vi "ShooterOutput.vi"() -> ()   [LabVIEW 2019]
uses:
  <vilib>/Rock Robotics/WPI/ThirdParty/REV Robotics/SPARK MAX/Typedef/Spark MAX Control Type.ctl
  <vilib>/Rock Robotics/WPI/Solenoid/WPI_SolenoidValue.ctl
  967c0bfc-6427-4b0b-9d33-318ccee3f8f4.vi
  ee6d7eed-3121-4b7e-b0b1-4827d4be6c14.vi
  refnums.vi
  GRNF_GenericMotor.vi
  GRNF_GenericSolenoid.vi
  sensors.vi
  outputs.vi
  dsdata.vi
  <vilib>/Rock Robotics/WPI/Solenoid/WPI_SolenoidSetEnum.vi
panel:
  in  "Plot Kicker":bool
  out "Kicker":T1(graph)
  in  "Kicker PID":T2={"P Gain"=0.0001, "I Gain"=1e-07, "D Gain"=0.01, "F Gain"=0.0002, "I Zone"=200.0, "Min Output"=0.0, "Max Output"=1.0} {"Max Output" min=-1.0 max=1.0 step=0.01; "Min Output" min=-1.0 max=1.0 step=0.01; "I Zone" step=0.01; "F Gain" step=0.01; "D Gain" step=0.01; "I Gain" step=0.01; "P Gain" min=0.0 step=0.01}
  out "Shooter 1":T1(graph)
  in  "Plot Shooter":bool
  out "Shooter 0":T1(graph)
  in  "Shooter PID":T2={"P Gain"=0.0027, "I Gain"=0.0, "D Gain"=0.007, "F Gain"=0.00017, "I Zone"=200.0, "Min Output"=0.0, "Max Output"=1.0} {"Max Output" min=-1.0 max=1.0 step=0.01; "Min Output" min=-1.0 max=1.0 step=0.01; "I Zone" step=0.01; "F Gain" step=0.01; "D Gain" step=0.01; "I Gain" step=0.01; "P Gain" min=0.0 step=0.01}
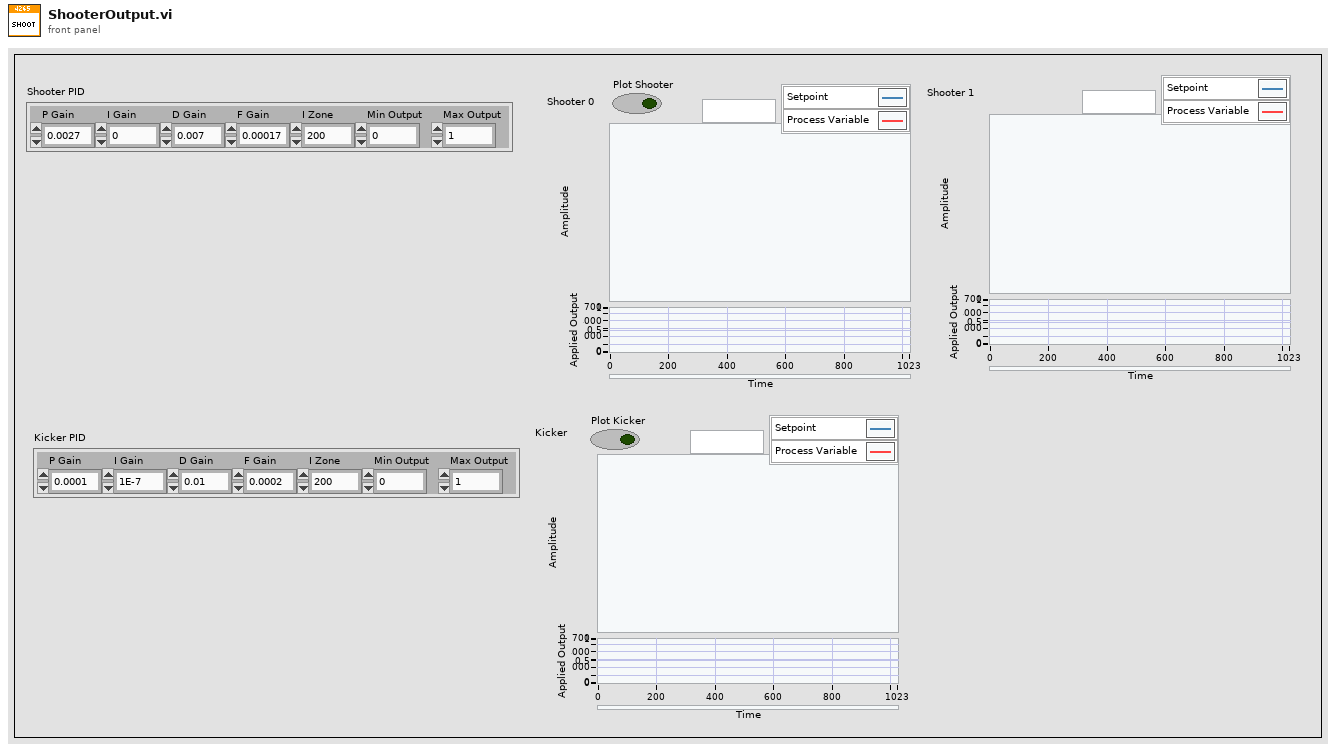
[diagram p1: front panel]
types:
  T1 = cluster{"Sensor Velocity":dbl, "Setpoint":dbl, "Applied Output":dbl}
  T2 = cluster{"P Gain":dbl, "I Gain":dbl, "D Gain":dbl, "F Gain":dbl, "I Zone":dbl, "Min Output":dbl, "Max Output":dbl}
  T3 = typedef "Spark MAX Control Type.ctl" = enum16{"Percent VBus", "Voltage", "Velocity", "Position", "Smart Motion", "Current", "Smart Velocity"}
  T4 = typedef "WPI_MotorControlDeviceRef.ctl" = cluster{"DeviceStatus":errorcluster, "Type":T5, "PWM":cluster{"PWM Channel":T6, "DeadBand":T7}, "CAN":cluster{"Device Number":u8, "SetOutput VI Ref":variant, "GetOutput VI Ref":variant, "Enable VI Ref":variant, "Disable VI Ref":variant, "Data":variant}, "Invert":bool, "DIO PWM":cluster{"PWM \"Enable\" Channel":T6, "DIOChannel":T8, "PWM Rate":dbl}}
  T5 = typedef "WPI_MotorControlType.ctl" = enum16{"PWM", "CAN", "DIO PWM"}
  T6 = typedef "FPGA_DIOPWMChannel.ctl" = enum8{"PWM 0", "PWM 1", "PWM 2", "PWM 3", "PWM 4", "PWM 5", "PWM 6", "PWM 7", "PWM 8", "PWM 9", "PWM MXP 0", "PWM MXP 1", "PWM MXP 2", "PWM MXP 3", "PWM MXP 4", "PWM MXP 5", "PWM MXP 6", "PWM MXP 7", "PWM MXP 8", "PWM MXP 9", "Invalid"}
  T7 = typedef "WPI_PWMDeadband.ctl" = cluster{"Name":string, "maxPositivePwm":i32, "minPositivePwm":i32, "centerPwm":i32, "maxNegativePwm":i32, "minNegativePwm":i32, "angularRange":u16}
  T8 = typedef "FPGA_DIOChannel.ctl" = enum8{"DIO 0", "DIO 1", "DIO 2", "DIO 3", "DIO 4", "DIO 5", "DIO 6", "DIO 7", "DIO 8", "DIO 9", "DIO MXP 0", "DIO MXP 1", "DIO MXP 2", "DIO MXP 3", "DIO MXP 4", "DIO MXP 5", "DIO MXP 6", "DIO MXP 7", "DIO MXP 8", "DIO MXP 9", "DIO MXP 10", "DIO MXP 11", "DIO MXP 12", "DIO MXP 13", "DIO MXP 14", "DIO MXP 15", "SPI Port CS1", "SPI Port CS2", "SPI Port CS3", "SPI Port MISO", "SPI Port MOSI", "Invalid"}
  T9 = typedef "WPI_SolenoidDevRef.ctl" = cluster{"DevStatus":errorcluster, "Pneumatics Control Module":u8, "Forward Solenoid Channel":T10, "Reverse Solenoid Channel":T10}
  T10 = typedef "WPI_SolenoidChannel.ctl" = enum8{"Solenoid 0", "Solenoid 1", "Solenoid 2", "Solenoid 3", "Solenoid 4", "Solenoid 5", "Solenoid 6", "Solenoid 7", "Invalid"}
  T11 = typedef "WPI_DriverStationRobotMode2.ctl" = enum16{"Autonomous Disabled", "Autonomous Enabled", "Teleop Disabled", "Teleop Enabled", "Disconnected", "Finish", "Test Disabled", "Test Enabled", "Emergency Stopped"}
  T12 = cluster{"P Gain":bool, "I Gain":bool, "D Gain":bool, "F Gain":bool, "I Zone":bool, "Min Output":bool, "Max Output":bool}
  T13 = typedef "WPI_SolenoidValue.ctl" = enum16{"Off", "On", "Forward", "Reverse"}
  T14 = cluster{"Goal_Kicker_Speed (rpm)":dbl, "Kicker_Velocity (rpm)":dbl, "Applied Output":dbl}
  T15 = cluster{"Goal_Shooter_Speed (rpm)":dbl, "Shooter_0_Velocity (rpm)":dbl, "Applied Output":dbl}
  T16 = cluster{"Goal_Shooter_Speed (rpm)":dbl, "Shooter_1_Velocity (rpm)":dbl, "Applied Output":dbl}
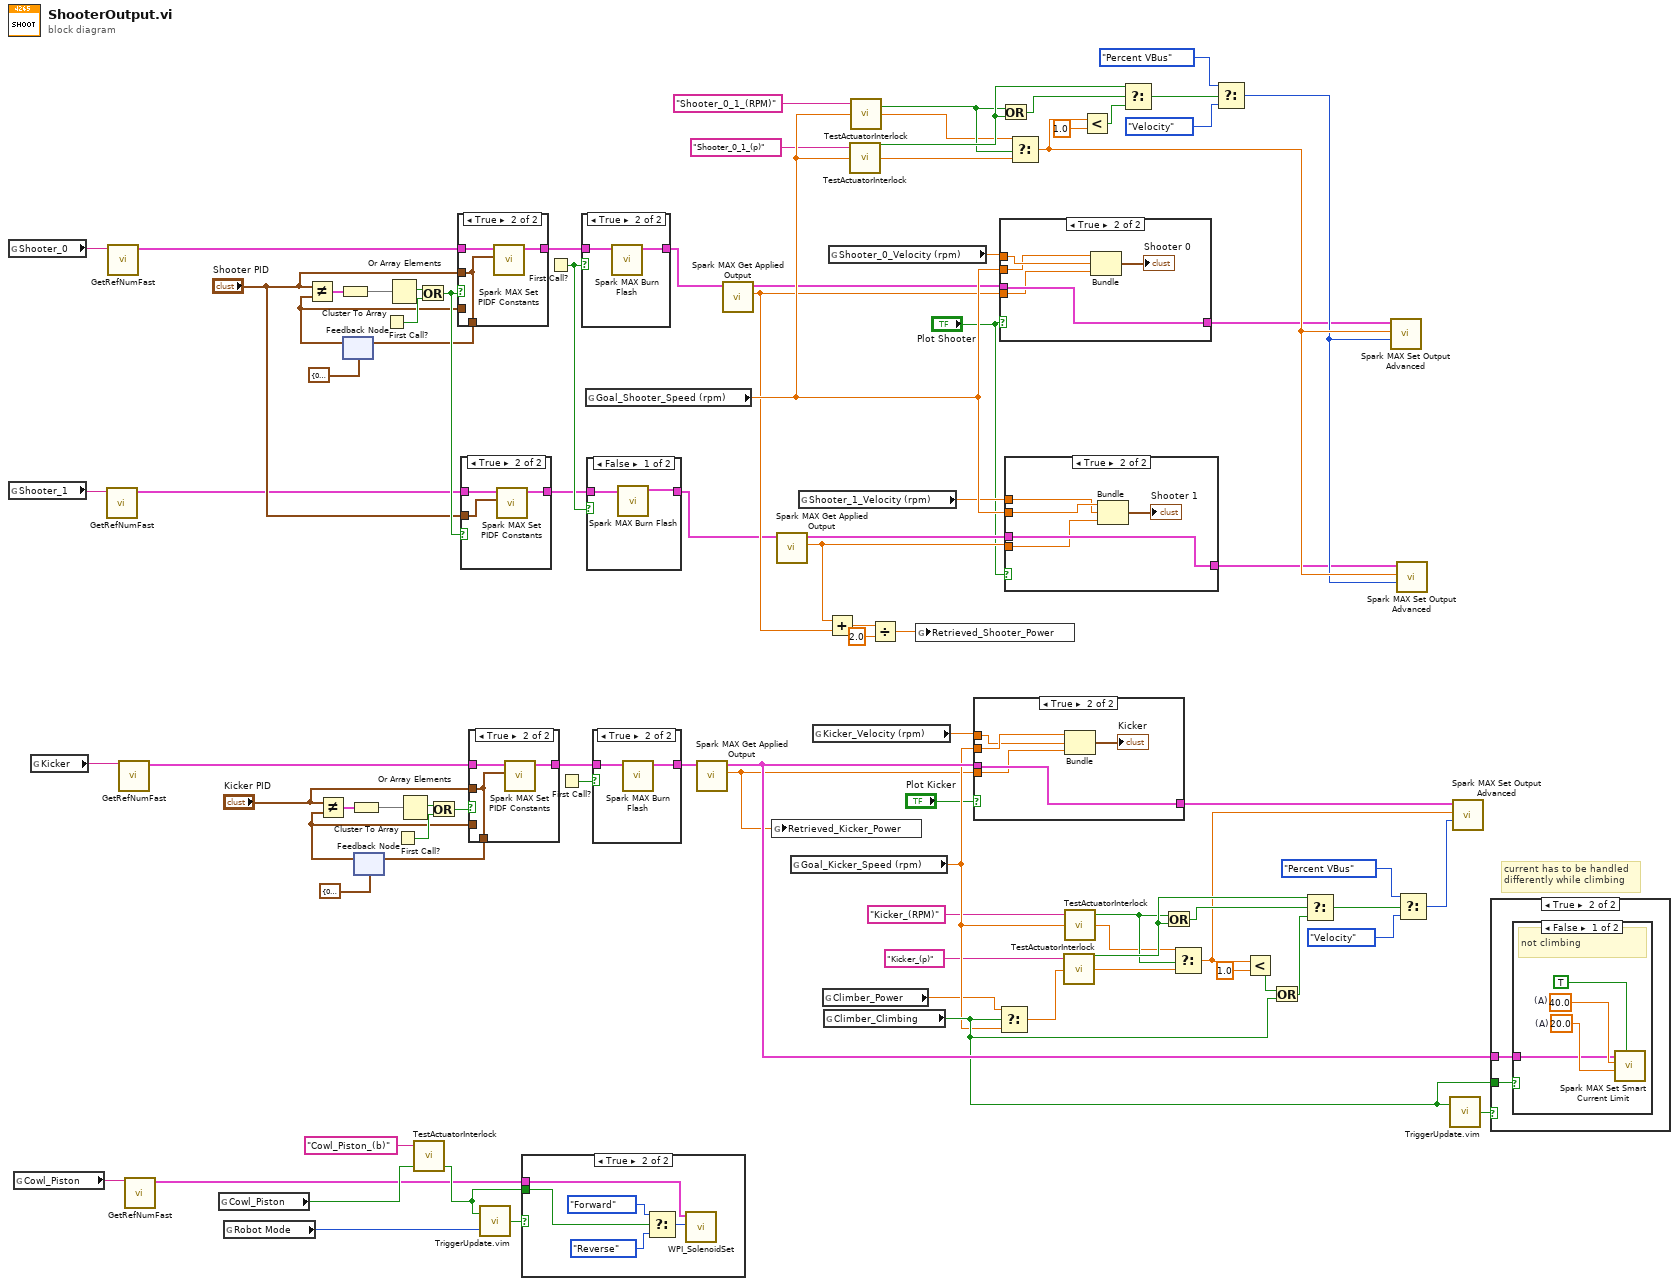
[diagram p0: block diagram]
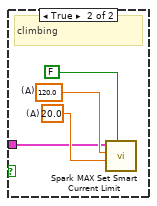
[diagram p3: hidden frame]
diagram:
  # "current has to be handled\ndifferently while climbing"
  n1 = global read "refnums.vi" "Shooter_0"() -> (w4:string)
  n2 = global read "refnums.vi" "Shooter_1"() -> (w3:string)
  n3 = global read "refnums.vi" "Cowl_Piston"() -> (w1:string)
  n4 = global read "refnums.vi" "Kicker"() -> (w2:string)
  n5 = call-poly "GetRefNumFast.vi"("RefNum Name"=w3) -> ("Device Reference"=w7:T4)  [unwired: 5 in, 1 out]
  n6 = call-poly "GetRefNumFast.vi"("RefNum Name"=w4) -> ("Device Reference"=w8:T4)  [unwired: 5 in, 1 out]
  n7 = call-poly "GetRefNumFast.vi"("RefNum Name"=w2) -> ("Device Reference"=w6:T4)  [unwired: 5 in, 1 out]
  n8 = call-poly "GetRefNumFast.vi"("RefNum Name"=w1) -> ("Device Reference"=w5:T9)  [unwired: 5 in, 1 out]
  n9 = global read "outputs.vi" "Cowl_Piston"() -> (w58:bool)
  n10 = global read "dsdata.vi" "Robot Mode"() -> (w35:T11)
  n11 = feedback #1(T2 {"P Gain"=0.0, "I Gain"=0.0, "D Gain"=0.0, "F Gain"=0.0, "I Zone"=0.0, "Min Output"=0.0, "Max Output"=0.0} ("PID Constants")) -> (w9:T2)
  n12 = Not Equal?(x="Shooter PID", y=w9) -> (x != y?=w13:T12)
  n13 = Cluster To Array(cluster=w13) -> (array=w12:bool[])
  n14 = feedback #2(T2 {"P Gain"=0.0, "I Gain"=0.0, "D Gain"=0.0, "F Gain"=0.0, "I Zone"=0.0, "Min Output"=0.0, "Max Output"=0.0} ("PID Constants")) -> (w37:T2)
  n15 = Not Equal?(x="Kicker PID", y=w37) -> (x != y?=w41:T12)
  n16 = Cluster To Array(cluster=w41) -> (array=w40:bool[])
  n17 = First Call?() -> (First Call?: T/F=w16:bool)
  n18 = Or Array Elements(Boolean array=w12) -> (logical OR=w15:bool)
  n19 = First Call?() -> (First Call?: T/F=w44:bool)
  n20 = Or Array Elements(Boolean array=w40) -> (logical OR=w43:bool)
  n21 = call "TestActuatorInterlock.vi"("Input_Value_Boolean"=w58, "Actuator_Name"="Cowl_Piston_(b)") -> ("Output_Value_Boolean"=w59:bool)  [unwired: 1 in, 2 out]
  n22 = Or(x=w15, y=w16) -> (x .or. y?=w19:bool)
  n23 = Or(x=w43, y=w44) -> (x .or. y?=w46:bool)
  n24 = case shown="True" w19 {
    tunnel: w8 -> [w92 w96]
    tunnel: "Shooter PID" -> [_ w94]
    tunnel: [w93 w94] -> w10
    tunnel: w9 -> [w93 _]
    tunnel: [w92 w95] -> w14
    frame False {
    }
    frame True {
      n25 = call <vilib>:"Spark MAX Set PIDF Constants.vi"("PID Constants"=w94, "MotorControlDeviceRef"=w96) -> ("MotorControlDeviceRef"=w95:T4)  [unwired: 8 in, 1 out]
    }
  }
  n26 = feedback-in #1(w10) -> ()
  n27 = case shown="True" w19 {
    tunnel: w7 -> [w97 w100]
    tunnel: "Shooter PID" -> [_ w98]
    tunnel: [w97 w99] -> w17
    frame False {
    }
    frame True {
      n28 = call <vilib>:"Spark MAX Set PIDF Constants.vi"("PID Constants"=w98, "MotorControlDeviceRef"=w100) -> ("MotorControlDeviceRef"=w99:T4)  [unwired: 8 in, 1 out]
    }
  }
  n29 = case shown="True" w46 {
    tunnel: w6 -> [w101 w105]
    tunnel: "Kicker PID" -> [_ w103]
    tunnel: [w102 w103] -> w38
    tunnel: w37 -> [w102 _]
    tunnel: [w101 w104] -> w42
    frame False {
    }
    frame True {
      n30 = call <vilib>:"Spark MAX Set PIDF Constants.vi"("PID Constants"=w103, "MotorControlDeviceRef"=w105) -> ("MotorControlDeviceRef"=w104:T4)  [unwired: 8 in, 1 out]
    }
  }
  n31 = feedback-in #2(w38) -> ()
  n32 = call "TriggerUpdate.vim"("Robot Mode"=w35, "Trigger"=w59) -> ("Update"=w36:bool)
  n33 = case shown="True" w36 {
    tunnel: w59 -> [_ w106]
    tunnel: w5 -> [_ w107]
    frame False {
    }
    frame True {
      n34 = Select(t=WPI_SolenoidValue."Forward" ("Value"), s=w106, f=WPI_SolenoidValue."Reverse" ("Value")) -> (s? t:f=w110:T13)
      n35 = call-poly <vilib>:"WPI_SolenoidSet.vi"("Value"=w110, "SolenoidDevRef"=w107) -> ()  [unwired: 8 in, 2 out]
    }
  }
  n36 = First Call?() -> (First Call?: T/F=w20:bool)
  n37 = First Call?() -> (First Call?: T/F=w47:bool)
  n38 = case shown="True" w20 {
    tunnel: w14 -> [w111 w113]
    tunnel: [w111 w112] -> w26
    frame False {
    }
    frame True {
      n39 = call <vilib>:"Spark MAX Burn Flash.vi"("MotorControlDeviceRef"=w113) -> ("MotorControlDeviceRef"=w112:T4)  [unwired: 9 in, 1 out]
    }
  }
  n40 = global read "outputs.vi" "Goal_Shooter_Speed (rpm)"() -> (w81:dbl)
  n41 = case shown="False" w20 {
    tunnel: [w114 w116] -> w28
    tunnel: w17 -> [w115 w116]
    frame False {
      n42 = call <vilib>:"Spark MAX Burn Flash.vi"("MotorControlDeviceRef"=w115) -> ("MotorControlDeviceRef"=w114:T4)  [unwired: 9 in, 1 out]
    }
    frame True {
    }
  }
  n43 = case shown="True" w47 {
    tunnel: w42 -> [w117 w119]
    tunnel: [w117 w118] -> w50
    frame False {
    }
    frame True {
      n44 = call <vilib>:"Spark MAX Burn Flash.vi"("MotorControlDeviceRef"=w119) -> ("MotorControlDeviceRef"=w118:T4)  [unwired: 9 in, 1 out]
    }
  }
  n45 = call <vilib>:"Spark MAX Get Applied Output.vi"("MotorControlDevRef in"=w50) -> ("Applied Output"=w56:dbl, "MotorControlDevRef out"=w91:T4)  [unwired: 7 in, 2 out]
  n46 = call <vilib>:"Spark MAX Get Applied Output.vi"("MotorControlDevRef in"=w26) -> ("Applied Output"=w31:dbl, "MotorControlDevRef out"=w27:T4)  [unwired: 7 in, 2 out]
  n47 = global write "sensors.vi" "Retrieved_Kicker_Power"(w56) -> ()
  n48 = call <vilib>:"Spark MAX Get Applied Output.vi"("MotorControlDevRef in"=w28) -> ("Applied Output"=w30:dbl, "MotorControlDevRef out"=w29:T4)  [unwired: 7 in, 2 out]
  n49 = global read "outputs.vi" "Goal_Kicker_Speed (rpm)"() -> (w85:dbl)
  n50 = global read "sensors.vi" "Shooter_1_Velocity (rpm)"() -> (w25:dbl)
  n51 = global read "sensors.vi" "Kicker_Velocity (rpm)"() -> (w49:dbl)
  n52 = global read "outputs.vi" "Climber_Power"() -> (w84:dbl)
  n53 = global read "outputs.vi" "Climber_Climbing"() -> (w90:bool)
  n54 = Add(x=w30, y=w31) -> (x+y=w32:dbl)
  n55 = global read "sensors.vi" "Shooter_0_Velocity (rpm)"() -> (w24:dbl)
  n56 = call "TestActuatorInterlock.vi"("Input_Value_Double"=w81, "Actuator_Name"="Shooter_0_1_(p)") -> ("Output_Value_Double"=w75:dbl, "In_Test_Mode"=w80:bool)  [unwired: 1 in, 1 out]
  n57 = call "TestActuatorInterlock.vi"("Input_Value_Double"=w81, "Actuator_Name"="Shooter_0_1_(RPM)") -> ("Output_Value_Double"=w74:dbl, "In_Test_Mode"=w76:bool)  [unwired: 1 in, 1 out]
  n58 = Divide(x=w32, y=2.0) -> (x/y=w34:dbl)
  n59 = global write "sensors.vi" "Retrieved_Shooter_Power"(w34) -> ()
  n60 = case shown="True" "Plot Kicker" {
    tunnel: w49 -> [_ w121]
    tunnel: w85 -> [_ w122]
    tunnel: w91 -> [w120 w124]
    tunnel: [w120 w124] -> w55
    tunnel: w56 -> [_ w123]
    frame False {
    }
    frame True {
      n61 = Bundle("Goal_Kicker_Speed (rpm)"=w122, "Kicker_Velocity (rpm)"=w121, "Applied Output"=w123) -> (→"Kicker":T14)  [unwired: 1 in]
    }
  }
  n62 = Select(t=w84, s=w90, f=w85) -> (s? t:f=w86:dbl)
  n63 = case shown="True" "Plot Shooter" {
    tunnel: w24 -> [_ w128]
    tunnel: w81 -> [_ w127]
    tunnel: w27 -> [w126 w130]
    tunnel: [w126 w130] -> w21
    tunnel: w31 -> [_ w129]
    frame False {
    }
    frame True {
      n64 = Bundle("Goal_Shooter_Speed (rpm)"=w127, "Shooter_0_Velocity (rpm)"=w128, "Applied Output"=w129) -> (→"Shooter 0":T15)  [unwired: 1 in]
    }
  }
  n65 = Or(x=w76, y=w80) -> (x .or. y?=w77:bool)
  n66 = case shown="True" "Plot Shooter" {
    tunnel: w25 -> [_ w133]
    tunnel: w29 -> [w132 w136]
    tunnel: w81 -> [_ w134]
    tunnel: [w132 w136] -> w22
    tunnel: w30 -> [_ w135]
    frame False {
    }
    frame True {
      n67 = Bundle("Goal_Shooter_Speed (rpm)"=w134, "Shooter_1_Velocity (rpm)"=w133, "Applied Output"=w135) -> (→"Shooter 1":T16)  [unwired: 1 in]
    }
  }
  n68 = Select(t=w74, s=w76, f=w75) -> (s? t:f=w83:dbl)
  n69 = call "TestActuatorInterlock.vi"("Input_Value_Double"=w86, "Actuator_Name"="Kicker_(p)") -> ("Output_Value_Double"=w63:dbl, "In_Test_Mode"=w68:bool)  [unwired: 1 in, 1 out]
  n70 = call "TestActuatorInterlock.vi"("Input_Value_Double"=w85, "Actuator_Name"="Kicker_(RPM)") -> ("Output_Value_Double"=w62:dbl, "In_Test_Mode"=w64:bool)  [unwired: 1 in, 1 out]
  n71 = Less?(x=w83, y=1.0) -> (x < y?=w78:bool)
  n72 = Select(t=w80, s=w77, f=w78) -> (s? t:f=w79:bool)
  n73 = Or(x=w64, y=w68) -> (x .or. y?=w66:bool)
  n74 = Select(t=w62, s=w64, f=w63) -> (s? t:f=w65:dbl)
  n75 = Select(t=Spark_MAX_Control_Type."Percent VBus" ("Control Mode"), s=w79, f=Spark_MAX_Control_Type."Velocity" ("Control Mode")) -> (s? t:f=w82:T3)
  n76 = Less?(x=w65, y=1.0) -> (x < y?=w87:bool)
  n77 = Or(x=w87, y=w90) -> (x .or. y?=w88:bool)
  n78 = Select(t=w68, s=w66, f=w88) -> (s? t:f=w67:bool)
  n79 = call <vilib>:"Spark MAX Set Output Advanced.vi"("Control Mode"=w82, "Setpoint"=w83, "MotorControlDevRef"=w21) -> ()  [unwired: 7 in, 2 out]
  n80 = call <vilib>:"Spark MAX Set Output Advanced.vi"("Control Mode"=w82, "Setpoint"=w83, "MotorControlDevRef"=w22) -> ()  [unwired: 7 in, 2 out]
  n81 = Select(t=Spark_MAX_Control_Type."Percent VBus" ("Control Mode"), s=w67, f=Spark_MAX_Control_Type."Velocity" ("Control Mode")) -> (s? t:f=w54:T3)
  n82 = call "TriggerUpdate.vim"("Trigger"=w90) -> ("Update"=w89:bool)  [unwired: 1 in]
  n83 = call <vilib>:"Spark MAX Set Output Advanced.vi"("Control Mode"=w54, "Setpoint"=w65, "MotorControlDevRef"=w55) -> ()  [unwired: 7 in, 2 out]
  n84 = case shown="True" w89 {
    tunnel: w90 -> [_ w139]
    tunnel: w91 -> [_ w138]
    frame False {
    }
    frame True {
      n85 = case shown="False" w139 {
        tunnel: w138 -> [w140 w144]
        frame False {
          w141 = 40.0  # (A)
          w142 = 20.0  # (A)
          # "not climbing"
          n86 = call <vilib>:"Spark MAX Set Smart Current Limit.vi"("Linearized Limit Enabled (F)"=TRUE, "Free Speed Current Limit (20A)"=w142, "Primay Current Limit (80A)"=w141, "MotorControlDeviceRef in"=w140) -> ()  [unwired: 6 in, 2 out]
        }
        frame True {
          w145 = 120.0  # (A)
          w146 = 20.0  # (A)
          # "climbing"
          n87 = call <vilib>:"Spark MAX Set Smart Current Limit.vi"("Linearized Limit Enabled (F)"=FALSE, "Free Speed Current Limit (20A)"=w146, "Primay Current Limit (80A)"=w145, "MotorControlDeviceRef in"=w144) -> ()  [unwired: 6 in, 2 out]
        }
      }
    }
  }
